vi "TestLUTBased.vi"() -> ()   [LabVIEW 2011]
uses:
  JelmersTracker.llb/TrackerDLL.vi
panel:
  in  "Photoncount / pixel":dbl(slide) scale=100.0..100000.0
  in  "Z":dbl(slide) min=0.0 max=99.0 scale=0.0..99.0
  in  "ZLUT radius":sgl=50.0
  out "Result":sgl[][](graph)
  in  "Position":cluster{"X":sgl, "Y":sgl}={"X"=125.0, "Y"=100.0}
  in  "Image Size":cluster{"Width":i32, "Height":i32}={"Width"=250, "Height"=200}
  out "LUT":u16[][](graph)
  in  "stop":bool
  in  "LUT original magnification":dbl=25.0
  in  "LUT image file":path=path "D:/jcnossen1/cudaqi-tracker/bin/LUTexample25X.jpg"
  out "Loop count":i32
  out "FPS":dbl
  in  "jump period":i32=20
  in  "x scalefactor":sgl=0.1
  in  "Z random factor":dbl
  in  "Use debug library":bool=TRUE
  out "appended path":path
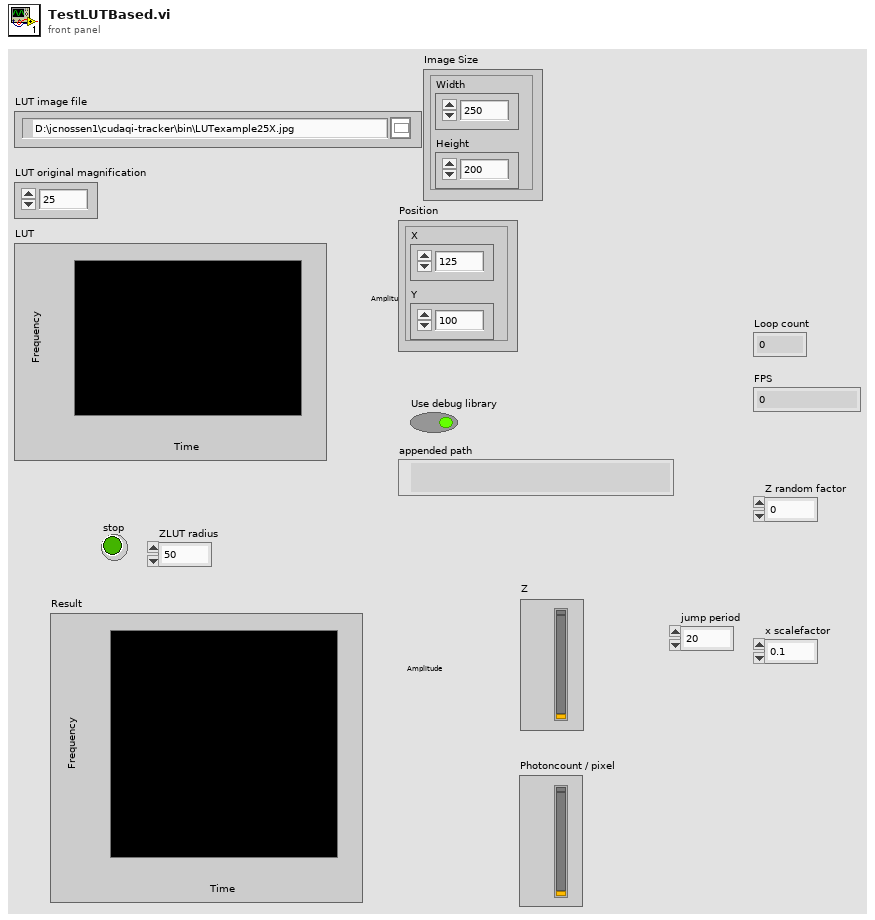
[diagram p1: front panel]
types:
  T1 = typedef "Image Type" = u32
  T2 = typedef "IMAQ Image.ctl" = refnum<image>
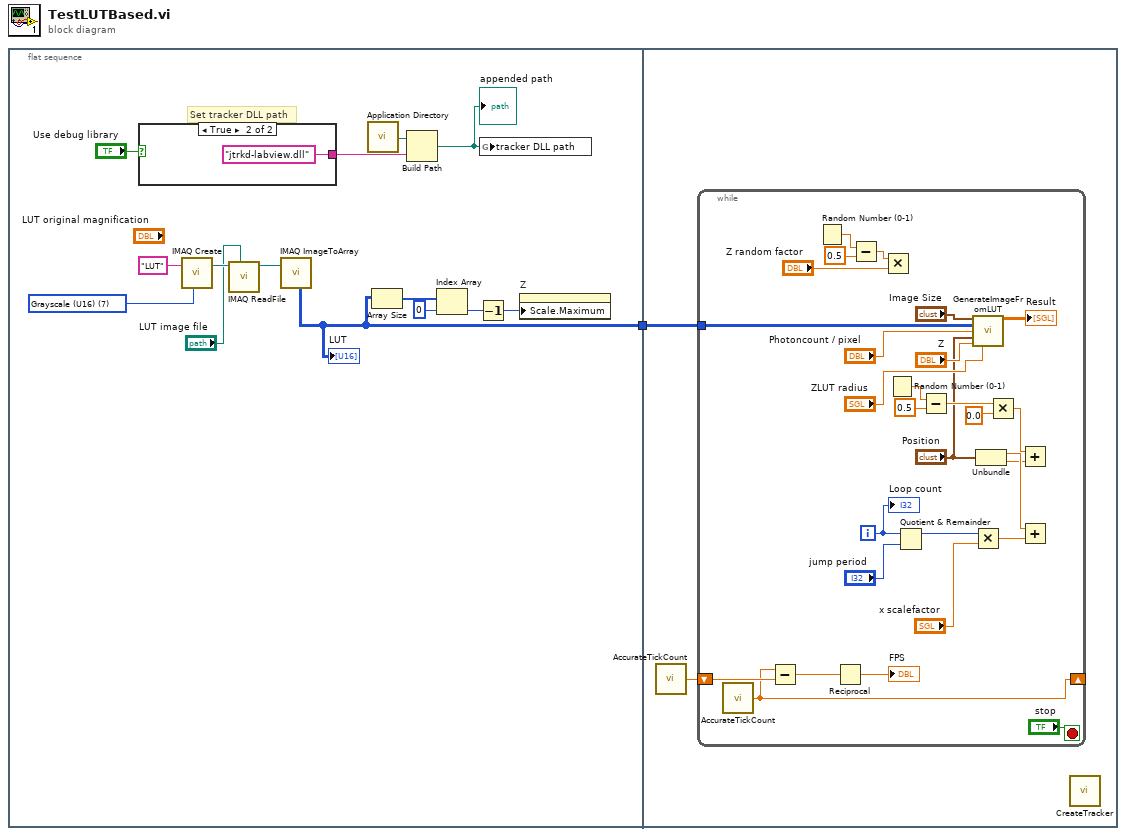
[diagram p0: block diagram]
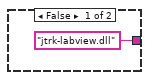
[diagram p2: hidden frame]
diagram:
  n1 = flat-sequence {
    tunnel: [w6] -> w1
    tunnel: w1 -> [w18]
    frame #0 {
      w11 = T1 7 items=["Grayscale (U8)", "Grayscale (I16)", "Grayscale (SGL)", "Complex (CSG)", "RGB (U32)", "HSL (U32)", "RGB (U64)", "Grayscale (U16)"] ("Image Type")
      # "Set tracker DLL path"
      n2 = case shown="True" "Use debug library" {
        tunnel: ["jtrk-labview.dll" "jtrkd-labview.dll"] -> w13
        frame False {
        }
        frame True {
        }
      }
      n3 = call "IMAQ Create"("Image Name"="LUT" ("String"), "Image Type"=w11) -> ("New Image"=w9:T2)  [unwired: 3 in, 1 out]
      n4 = call "IMAQ ReadFile"("File Path"="LUT image file", "Image"=w9) -> ("Image Out"=w7:T2)  [unwired: 5 in, 4 out]
      n5 = call "IMAQ ImageToArray"("Image"=w7) -> ("Image Pixels (U16)"=w6:u16[][])  [unwired: 3 in, 4 out]
      "LUT" <- w6
      n6 = call <vilib>:"Application Directory.vi"() -> ("Application Directory"=w12:path)
      n7 = Array Size(array=w6) -> (size(s)=w5:i32[])
      n8 = Build Path(base path=w12, name or relative path=w13) -> (appended path=w14:path)
      "appended path" <- w14
      n9 = Index Array(array=w5, index=0) -> (element=w3:i32)
      n10 = Decrement(x=w3) -> (x-1=w2:i32)
      n11 = global write "TrackerDLL.vi" "tracker DLL path"(w14) -> ()
      n12 = property on="Z" class="Slide (strict)"("Scale.Maximum"=w2) -> ()  [unwired: 2 in, 2 out]
    }
    frame #1 {
      n13 = call "AccurateTickCount.vi"() -> ("seconds"=w19:dbl)
      n14 = while {
        shift-right: [w42] -> _
        shift-left: w19 -> [w43]
        tunnel: w18 -> [w24]
        i -> [w39]
        stop <- "stop" stop-if-true
        n15 = call "AccurateTickCount.vi"() -> ("seconds"=w42:dbl)
        n16 = Subtract(x=w42, y=w43) -> (x-y=w41:dbl)
        n17 = Random Number (0-1)() -> (number: 0 to 1=w33:dbl)
        n18 = Reciprocal(x=w41) -> (1/x=→"FPS":dbl)
        n19 = Subtract(x=w33, y=0.5) -> (x-y=w31:dbl)
        n20 = Multiply(x=w31, y="Z random factor") -> ()  [unwired: 1 out]
        n21 = Random Number (0-1)() -> (number: 0 to 1=w46:dbl)
        n22 = Quotient & Remainder(x=w39, y="jump period") -> (x-y*floor(x/y)=w37:i32)  [unwired: 1 out]
        n23 = Subtract(x=w46, y=0.5) -> (x-y=w44:dbl)
        n24 = call "GenerateImageFromLUT.vi"("Image Size"="Image Size", "ZLUT"=w24, "Photon count / pixel"="Photoncount / pixel", "Position"="Position", "zpos"="Z", "ZLUT radius"="ZLUT radius") -> ("Result image"=→"Result":sgl[][])  [unwired: 9 in]
        n25 = Multiply(x=w37, y="x scalefactor") -> (x*y=w35:sgl)
        n26 = Unbundle("Position") -> ("X"=w28:sgl, "Y"=w27:sgl)
        n27 = Multiply(x=w44, y=sgl 0.0) -> (x*y=w47:dbl)
        n28 = Add(x=w47, y=w27) -> ()  [unwired: 1 out]
        n29 = Add(x=w28, y=w35) -> ()  [unwired: 1 out]
        "Loop count" <- w39
      }
      n30 = call "CreateTracker.vi"() -> ()  [unwired: 3 in, 1 out]
    }
  }
